vi "NanotecSMCPDDriver.transaction.vi"(0 "VISAresource":refnum<visa-resource-name>, 1 "contollerID":i32=-1, 2 "commandString":string, 3 "Bytes to read (1024)":u32=1024, 5 "error in (no error)":errorcluster) -> (14 "VISAresource out":refnum<visa-resource-name>, 15 "contollerID out":i32=-1, 16 "response":string, 17 "bytes read":i32, 18 "device  Errno":i32, 19 "error out":errorcluster)   [LabVIEW 2015, in "NanotecSMCPDDriver.lvlib"]
doc: "Makes the transaction with an Nanotec device, formating command or query strings, sends and reads strings, locks and unlocks the VISA source."
uses:
  NanotecSMCPDDriver.lvlib
panel:
  out "read buffer":string
  out "write buffer (\"\")":string
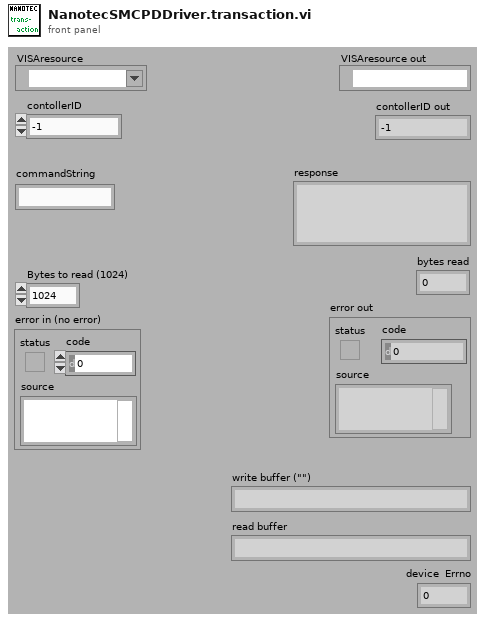
[diagram p1: front panel]
types:
  T1 = enum16{"unknown", "add", "remove", "get", "cleanup"}
  T2 = typedef "Semaphore RefNum" = refnum<k1>
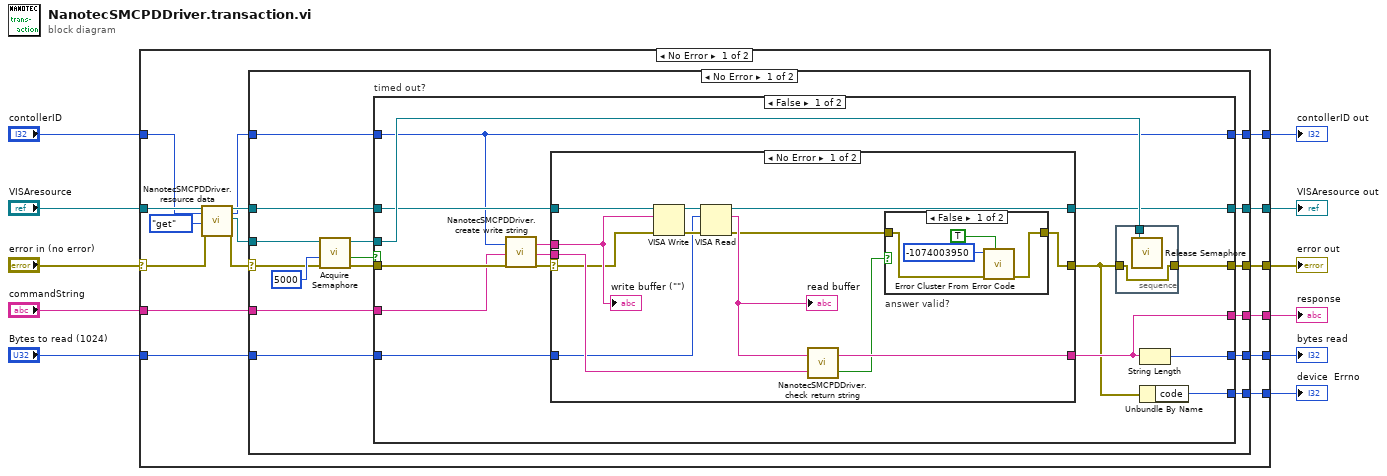
[diagram p0: block diagram]
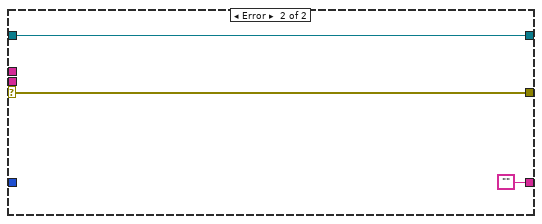
[diagram p3: hidden frame]
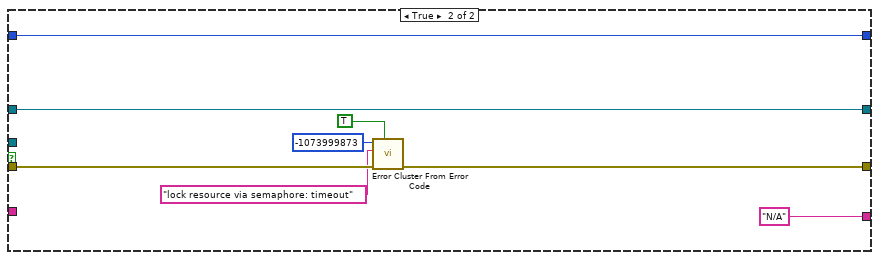
[diagram p4: hidden frame]
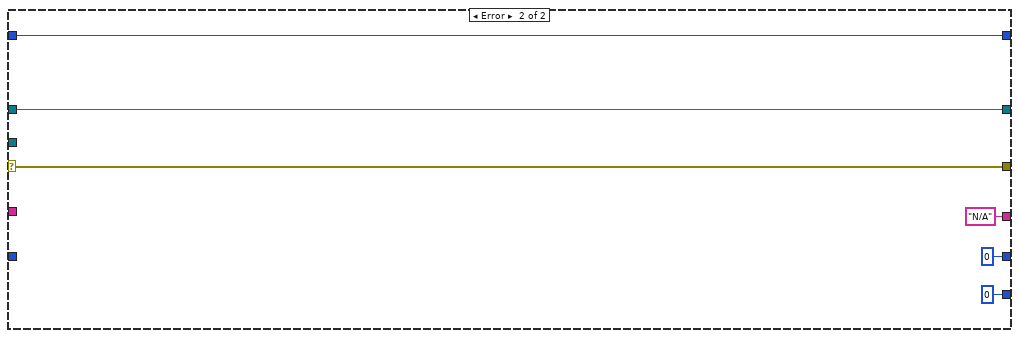
[diagram p5: hidden frame]
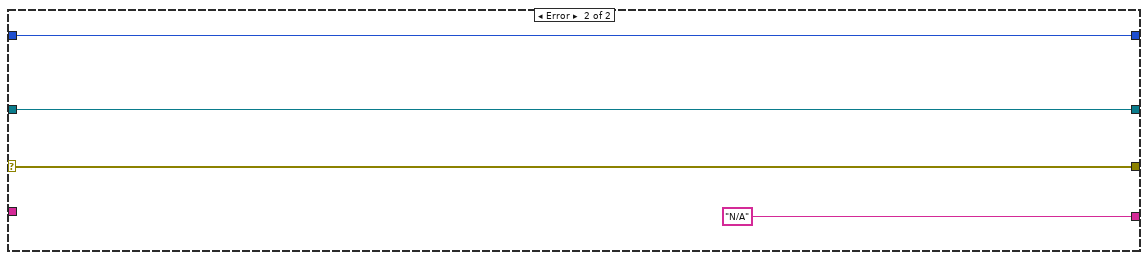
[diagram p6: hidden frame]
diagram:
  n1 = case shown="No Error" "error in (no error)" {
    selector: "error in (no error)" -> [w23 w99]
    tunnel: [w27 "N/A" ("data string")] -> w8
    tunnel: [w26 w99] -> w10
    tunnel: [w25 _] -> w9
    tunnel: [w24 _] -> w7
    tunnel: "VISAresource" -> [w21 w97]
    tunnel: "contollerID" -> [w20 w96]
    tunnel: [w17 w97] -> w4
    tunnel: [w16 w96] -> w3
    tunnel: "Bytes to read (1024)" -> [w13 _]
    tunnel: "commandString" -> [w12 _]
    frame No Error {
      n2 = call "NanotecSMCPDDriver.resource data.vi"("VISAresource"=w21, "contollerID"=w20, "action"=T1."get", "error in (no error)"=w23) -> ("VISAresource out"=w22:refnum<visa-resource-name>, "contollerID out"=w18:i32, "semaphore"=w19:T2, "error out"=w14:errorcluster)  [unwired: 11 in, 1 out]
      n3 = case shown="No Error" w14 {
        selector: w14 -> [w30 w93]
        tunnel: [w43 "N/A" ("data string")] -> w27
        tunnel: [w42 w93] -> w26
        tunnel: [w41 0 ("code")] -> w25
        tunnel: [w40 0] -> w24
        tunnel: w22 -> [w36 w94]
        tunnel: w19 -> [w35 _]
        tunnel: w18 -> [w34 w95]
        tunnel: [w33 w94] -> w17
        tunnel: [w32 w95] -> w16
        tunnel: w13 -> [w29 _]
        tunnel: w12 -> [w28 _]
        frame No Error {
          n4 = call <vilib>:"Acquire Semaphore.vi"("error in (no error)"=w30, "ms timeout (-1)"=5000, "semaphore"=w35) -> ("error out"=w39:errorcluster, "timed out"=w37:bool, "semaphore out"=w38:T2)  [unwired: 2 in]
          n5 = case "timed out?" shown="False" w37 {
            tunnel: [w49 "N/A" ("data string")] -> w43
            tunnel: [w55 w85] -> w42
            tunnel: [w58 _] -> w41
            tunnel: [w57 _] -> w40
            tunnel: w39 -> [w47 w88]
            tunnel: w38 -> [w56 _]
            tunnel: w36 -> [w54 w83]
            tunnel: w34 -> [w52 w82]
            tunnel: [w53 w83] -> w33
            tunnel: [w52 w82] -> w32
            tunnel: w29 -> [w45 _]
            tunnel: w28 -> [w44 _]
            frame False {
              n6 = call "NanotecSMCPDDriver.create write string.vi"("contollerID"=w52, "commandString"=w44, "error in (no error)"=w47) -> ("writeString"=w51:string, "expextedReturnString"=w50:string, "error out"=w46:errorcluster)  [unwired: 14 in]
              n7 = case shown="No Error" w46 {
                selector: w46 -> [w60 w79]
                tunnel: w54 -> [w69 w78]
                tunnel: [w68 w78] -> w53
                tunnel: w51 -> [w67 _]
                tunnel: w50 -> [w65 _]
                tunnel: [w64 "" ("Empty String Constant")] -> w49
                tunnel: [w61 w79] -> w48
                tunnel: w45 -> [w59 _]
                frame No Error {
                  n8 = VISA Write(VISA resource name=w69, write buffer=w67, error in (no error)=w60) -> (VISA resource name out=w70:refnum<visa-resource-name>, error out=w71:errorcluster)  [unwired: 1 out]
                  n9 = VISA Read(VISA resource name=w70, byte count=w59, error in (no error)=w71) -> (VISA resource name out=w68:refnum<visa-resource-name>, read buffer=w66:string, error out=w62:errorcluster)  [unwired: 1 out]
                  "read buffer" <- w66
                  n10 = call "NanotecSMCPDDriver.check return string.vi"("expextedReturnString"=w65, "readString"=w66) -> ("answerValid"=w63:bool, "string"=w64:string)
                  n11 = case "answer valid?" shown="False" w63 {
                    tunnel: w62 -> [w75 w76]
                    tunnel: [w74 w76] -> w61
                    frame False {
                      n12 = call <vilib>:"Error Cluster From Error Code.vi"("show call chain? (False)"=TRUE, "error in (no error)"=w75, "error code (0)"=-1074003950) -> ("error out"=w74:errorcluster)  [unwired: 6 in]
                    }
                    frame True {
                    }
                  }
                  "write buffer (\"\")" <- w67
                }
                frame Error {
                }
              }
              n13 = stacked-sequence {
                tunnel: w56 -> [w81]
                tunnel: [w80] -> w55
                tunnel: w48 -> [w80]
                frame #0 {
                  n14 = call <vilib>:"Release Semaphore.vi"("semaphore"=w81) -> ()  [unwired: 5 in, 2 out]
                }
              }
              n15 = String Length(string=w49) -> (length=w57:i32)
              n16 = Unbundle By Name(w48) -> ("code"=w58:i32)
            }
            frame True {
              n17 = call <vilib>:"Error Cluster From Error Code.vi"("show call chain? (False)"=TRUE, "error in (no error)"=w88, "error message (\"\")"="lock resource via semaphore: timeout" ("error message (\"\")"), "error code (0)"=-1073999873) -> ("error out"=w85:errorcluster)  [unwired: 5 in]
            }
          }
        }
        frame Error {
        }
      }
    }
    frame Error {
    }
  }
  "device  Errno" <- w9
  "response" <- w8
  "error out" <- w10
  "bytes read" <- w7
  "VISAresource out" <- w4
  "contollerID out" <- w3
